vi "Get Controls.vi"(8 "error in (no error)":errorcluster, 10 "Flex Msg in":refnum<class "Flex Msg.lvclass">, 11 "VI Refnum in":refnum<vi>) -> (0 "error out":errorcluster, 2 "Control Element Array":T1[](array[typedef]), 3 "VI Refnum out":refnum<vi>)   [LabVIEW 2020, in "Msg.lvlib" / "Flex Msg.lvclass"]
doc: "Get all controls and indicators from the front panel of 'VI Refnum in'. Only elements with labels not in 'Label Exclusions' that are visible and has a valid Control Index are returned."
uses:
  Flex Msg.lvclass
  Controls/Ctl_Control Element.ctl
  Msg.lvlib
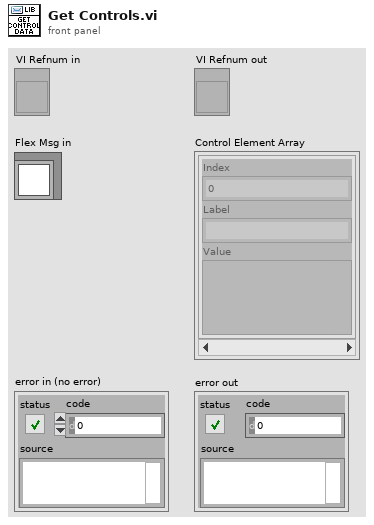
[diagram p1: front panel]
types:
  T1 = typedef "Msg.lvlib/Ctl_Control Element.ctl" = cluster{"Index":i32, "Label":string, "Value":variant}
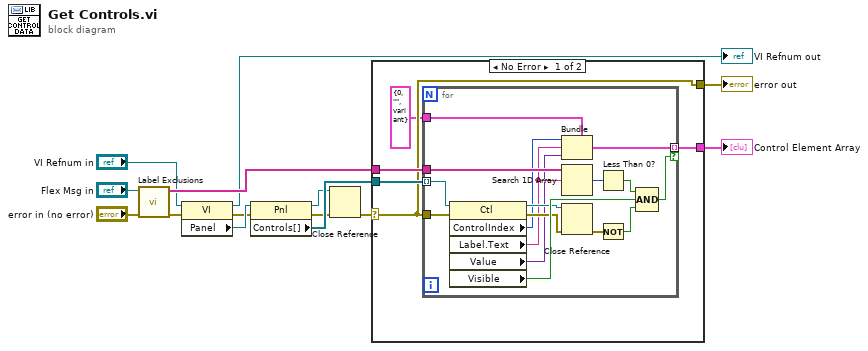
[diagram p0: block diagram]
diagram:
  n1 = call-dynamic "Label Exclusions.vi"("error in (no error)"="error in (no error)", "Flex Msg in"="Flex Msg in") -> ("error out"=w9:errorcluster, "Label Exclusions"=w11:string[])  [unwired: 8 in]
  n2 = property class="VI"(reference="VI Refnum in", error in=w9) -> (reference out=→"VI Refnum out":refnum<vi>, error out=w6:errorcluster, "Panel"=w14:refnum<vi>)
  n3 = property class="Pnl"(reference=w14, error in=w6) -> (reference out=w8:refnum<vi>, error out=w7:errorcluster, "Controls[]"=w13:refnum<vi>[])
  n4 = Close Reference(reference=w8, error in (no error)=w7) -> (error out=w5:errorcluster)
  n5 = case shown="No Error" w5 {
    selector: w5 -> [w16 w36]
    tunnel: w13 -> [w19 _]
    tunnel: w11 -> [w18 _]
    tunnel: [w17 _] -> w2
    tunnel: [w16 w36] -> w3
    frame No Error {
      n6 = for {
        tunnel: w19 -> [w35] mode=indexing
        tunnel: [w20] -> w17 mode=indexing if=w30
        tunnel: w18 -> [w34]
        tunnel: w16 -> [w25]
        tunnel: T1 {"Index"=0, "Label"="", "Value"=variant} ("Control element") -> [w24]
        n7 = property class="Ctl"(reference=w35, error in=w25) -> (reference out=w29:refnum<vi>, error out=w28:errorcluster, "ControlIndex"=w23:i32, "Label.Text"=w22:string, "Value"=w21:variant, "Visible"=w31:bool)
        n8 = Bundle(cluster=w24, "Index"=w23, "Label"=w22, "Value"=w21) -> (w20:T1)
        n9 = Search 1D Array(1D array=w34, element=w22) -> (index of element=w33:i32)  [unwired: 1 in]
        n10 = Close Reference(reference=w29, error in (no error)=w28) -> (error out=w27:errorcluster)
        n11 = Less Than 0?(x=w33) -> (x < 0?=w32:bool)
        n12 = Not(x=w27) -> (.not. x?=w26:bool)
        n13 = Compound Arithmetic op=AND(w32, w31, w26) -> (w30:bool)
      }
    }
    frame Error {
    }
  }
  "error out" <- w3
  "Control Element Array" <- w2
